vi "Step-3-hp_state-i.vi"(9 "hp_state_in (u64)":u64[](array[numeric]) format="%.0x", 11 "j":u64) -> (1 "U64-Array":u64[](array[numeric]) format="%.0x")   [LabVIEW 2017]
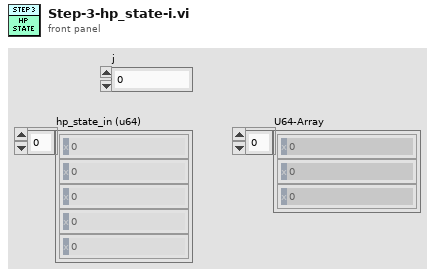
[diagram p1: front panel]
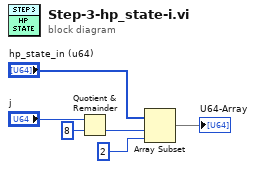
[diagram p0: block diagram]
diagram:
  n1 = Quotient & Remainder(x="j", y=u64 8) -> (floor(x/y)=w3:u64)  [unwired: 1 out]
  n2 = Array Subset(array="hp_state_in (u64)", index=w3, length=2) -> (→"U64-Array":u64[])
